vi "TestFastEncoder1.vi"() -> ()   [LabVIEW 2010]
uses:
  <vilib>/eio/EIONode/EIONode.xnode
  <vilib>/rvi/eio/nirviEIOImplementation/nirviEIOImplementation.xnode
  <vilib>/rvi/eio/common/nirviEmuClasses.ctl
  <vilib>/rvi/eio/common/nirviEmuTemplateMethod_noerrors.vi
panel:
  out "Steering Center":bool
  out "SteerEncoderA":bool
  out "SteerEncoderB":bool
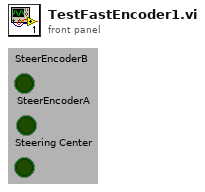
[diagram p1: front panel]
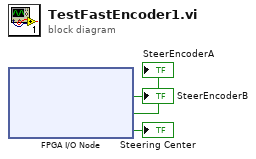
[diagram p0: block diagram]
diagram:
  n1 = xnode "FPGA I/O Node"() -> ("SteerEncoderB"=→"SteerEncoderB":bool, "SteerEncoderA"=→"SteerEncoderA":bool, "Steering Center"=→"Steering Center":bool)  [unwired: 3 in, 3 out]
